vi "gotoTopBotExp2.vi"(8 "error in (no error)":errorcluster, 9 "position":refnum<vi>, 10 "motor setting":refnum<vi>, 11 "appended array":refnum<k7>[](array[refnum])) -> (0 "error out":errorcluster)   [LabVIEW 2014]
panel:
  in  "bwait":bool
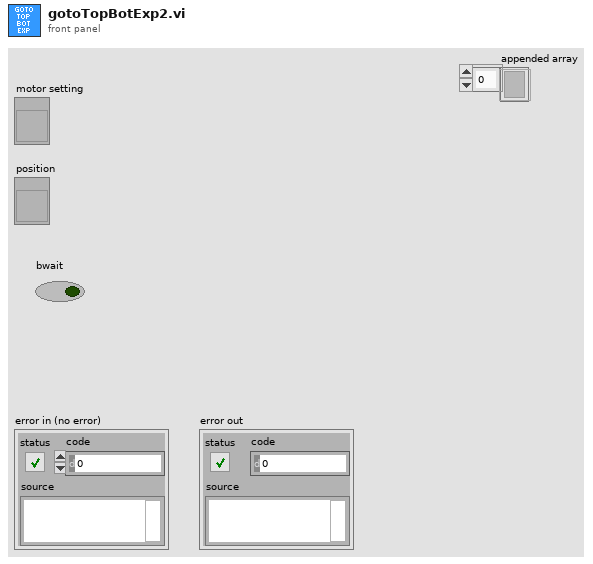
[diagram p1: front panel]
types:
  T1 = cluster{"X Acc (mm/s^2)":sgl, "X Vmax (mm/s)":sgl, "Y Acc (mm/s^2)":sgl, "Y Vmax (mm/s)":sgl, "Z Acc (mm/s^2)":sgl, "Z Vmax (mm/s)":sgl}
  T2 = cluster{"X Pos (mm)":sgl, "Y Pos (mm)":sgl, "Z Pos (mm)":sgl}
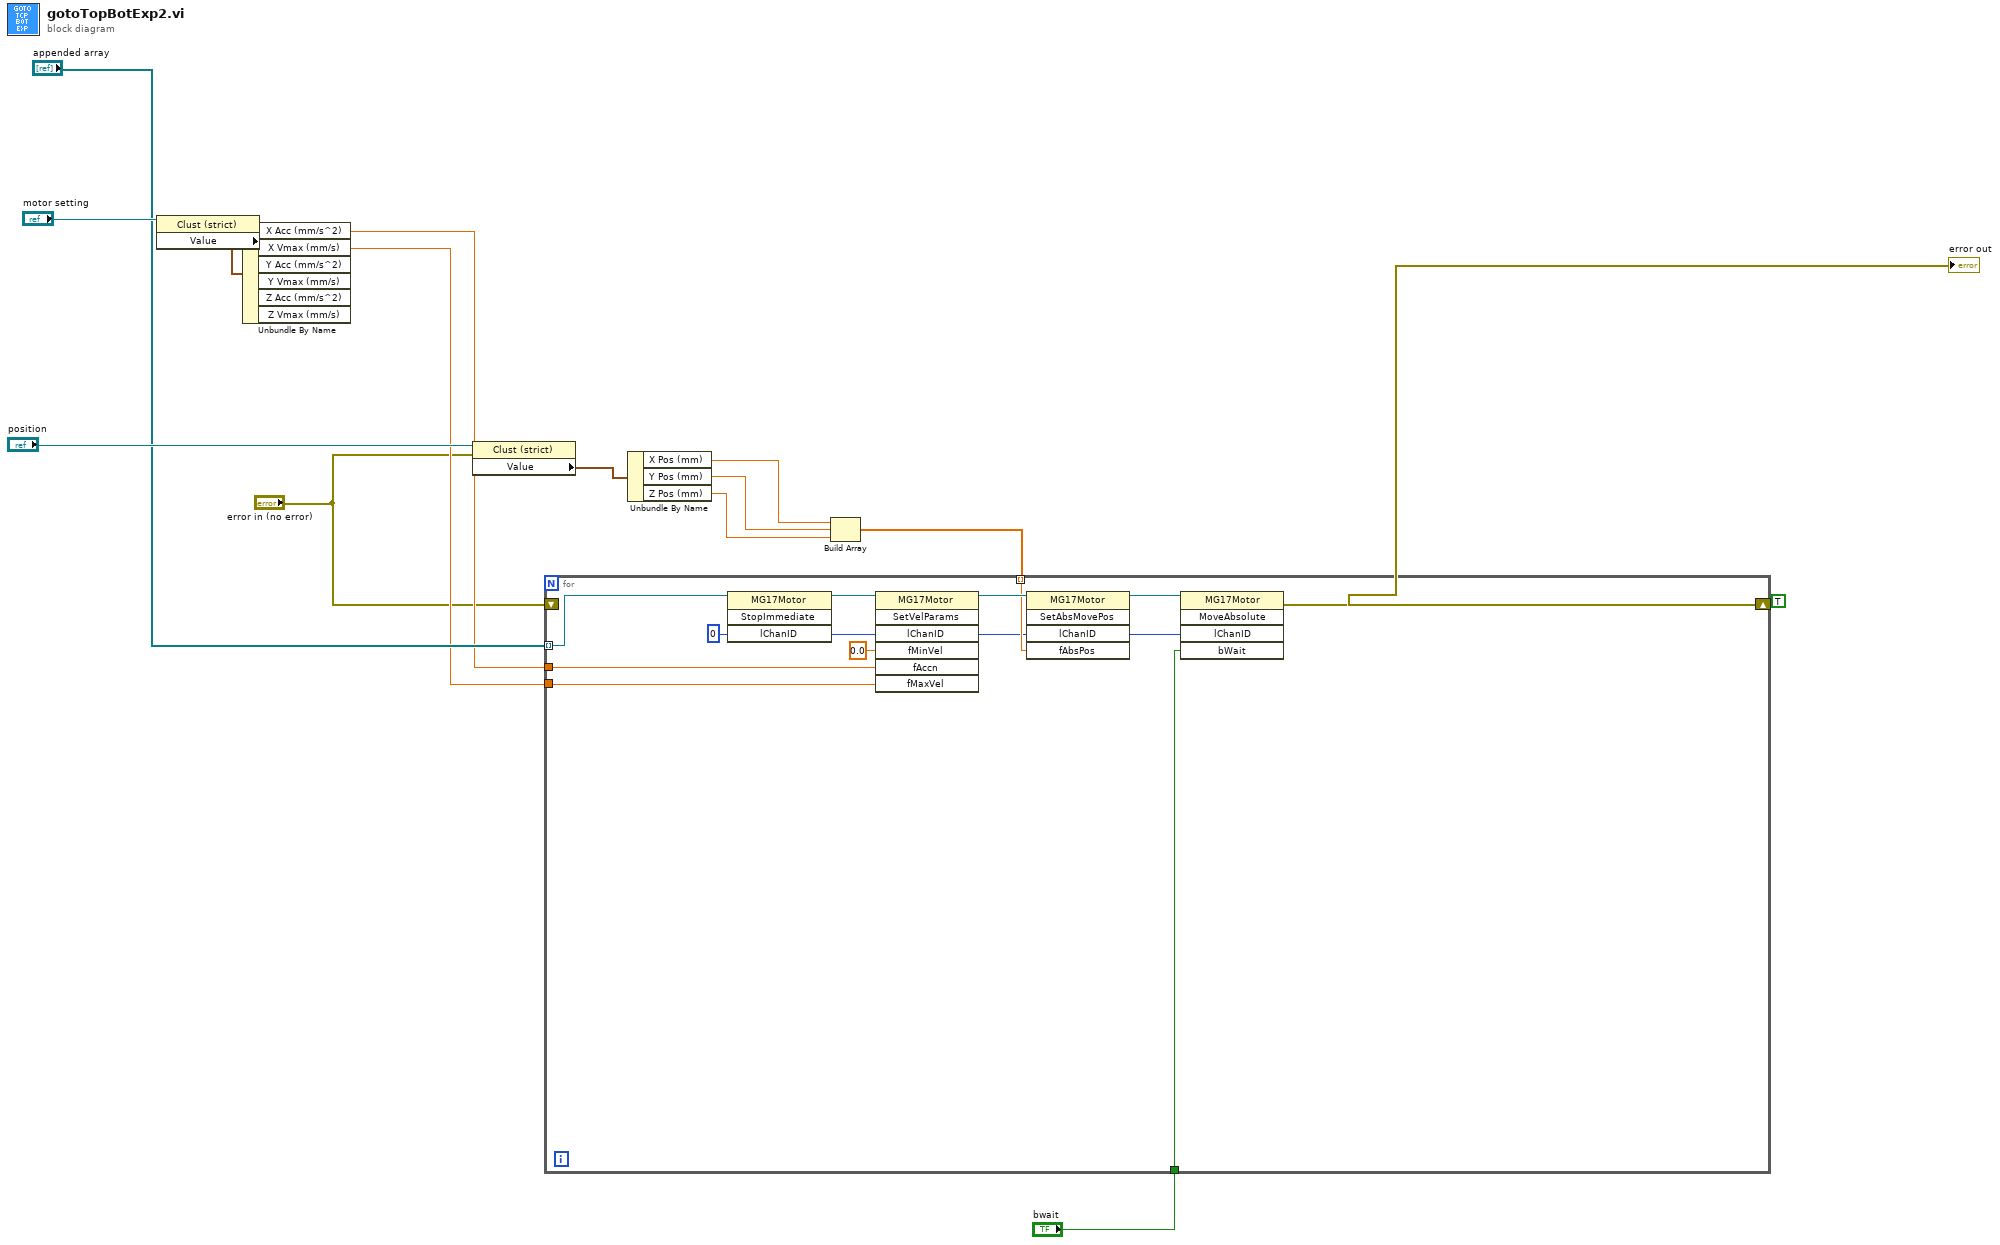
[diagram p0: block diagram]
diagram:
  (unwired) TRUE
  n1 = property on="Property Node" class="Clust (strict)"(reference="motor setting") -> ("Value"=w9:T1)  [unwired: 1 in, 2 out]
  n2 = Unbundle By Name(w9) -> ("X Acc (mm/s^2)"=w7:sgl, "X Vmax (mm/s)"=w8:sgl)  [unwired: 4 out]
  n3 = property on="Property Node" class="Clust (strict)"(reference="position", error in="error in (no error)") -> ("Value"=w10:T2)  [unwired: 2 out]
  n4 = Unbundle By Name(w10) -> ("X Pos (mm)"=w6:sgl, "Y Pos (mm)"=w5:sgl, "Z Pos (mm)"=w4:sgl)
  n5 = Build Array(w6, w5, w4) -> (w3:sgl[])
  n6 = for {
    tunnel: "appended array" -> [w28] mode=indexing
    tunnel: w8 -> [w22]
    tunnel: w7 -> [w21]
    tunnel: w3 -> [w19] mode=indexing
    shift-right: [w18] -> w14
    shift-left: "error in (no error)" -> [_]
    tunnel: "bwait" -> [w15]
    n7 = invoke class="MG17Motor" method="StopImmediate"(reference=w28, "lChanID"=0) -> (reference out=w27:refnum<k7>, "lChanID"=w17:i32)  [unwired: 2 in, 2 out]
    n8 = invoke class="MG17Motor" method="SetVelParams"(reference=w27, "lChanID"=w17, "fMinVel"=sgl 0.0, "fAccn"=w21, "fMaxVel"=w22) -> (reference out=w26:refnum<k7>, "lChanID"=w16:i32)  [unwired: 2 in, 5 out]
    n9 = invoke class="MG17Motor" method="SetAbsMovePos"(reference=w26, "lChanID"=w16, "fAbsPos"=w19) -> (reference out=w25:refnum<k7>, "lChanID"=w20:i32)  [unwired: 2 in, 3 out]
    n10 = invoke class="MG17Motor" method="MoveAbsolute"(reference=w25, "lChanID"=w20, "bWait"=w15) -> (error out=w18:errorcluster)  [unwired: 2 in, 4 out]
  }
  "error out" <- w14
